vi "Check for Valid File Paths.vi"(8 "error in":errorcluster, 10 "Input Paths (in)":T1={"Golden Template (Source) - (make relative)"=path "E:/Documents/Projects/SPIAPI/Pre-GitHub/Scripting Code 02_10_15 - Cleanup Time/IONode", "Destination Generated Code (make relative)"=path "E:/Documents/Projects/SPIAPI/Pre-GitHub/Scripting Code 02_10_15 - Cleanup Time/Test", "LabVIEW Project to Script"=path "E:/Documents/Projects/SPIAPI/Pre-GitHub/Scripting Code 02_10_15 - Cleanup Time/Test/Test.lvproj", "Placement VI"=path "E:/Documents/Projects/SPIAPI/Pre-GitHub/Scripting Code 02_10_15 - Cleanup Time/Test/TestVI.VI"}, 11 "State Queue In":refnum<queue>) -> (0 "error out":errorcluster, 2 "Inputs Paths (out)":T1={"Golden Template (Source) - (make relative)"=path "E:/Documents/Projects/SPIAPI/Scripting Code  with State Machine 01_12_15 - IO Node Control Still Needs Updating/IONode", "Destination Generated Code (make relative)"=path "E:/Documents/Projects/SPIAPI/Examples", "LabVIEW Project to Script"=path "E:/Documents/Projects/SPIAPI/Examples/SPI Engine Example.lvproj", "Placement VI"=path "E:/Documents/Projects/SPIAPI/Examples/PMOD Example(FPGA).vi"}, 3 "State Queue Out":refnum<queue>)   [LabVIEW 2014]
doc: "Checks if a file/ folder exists at all input paths. Throws an error if they don't. If the Placement VI is blank, change the path to point to Generated Code.vi and queue Generate FPGA VI state.s"
uses:
  Controls/Input Paths.ctl
  Scripting States.ctl
  Initialization and IO Node Scripting.lvlib
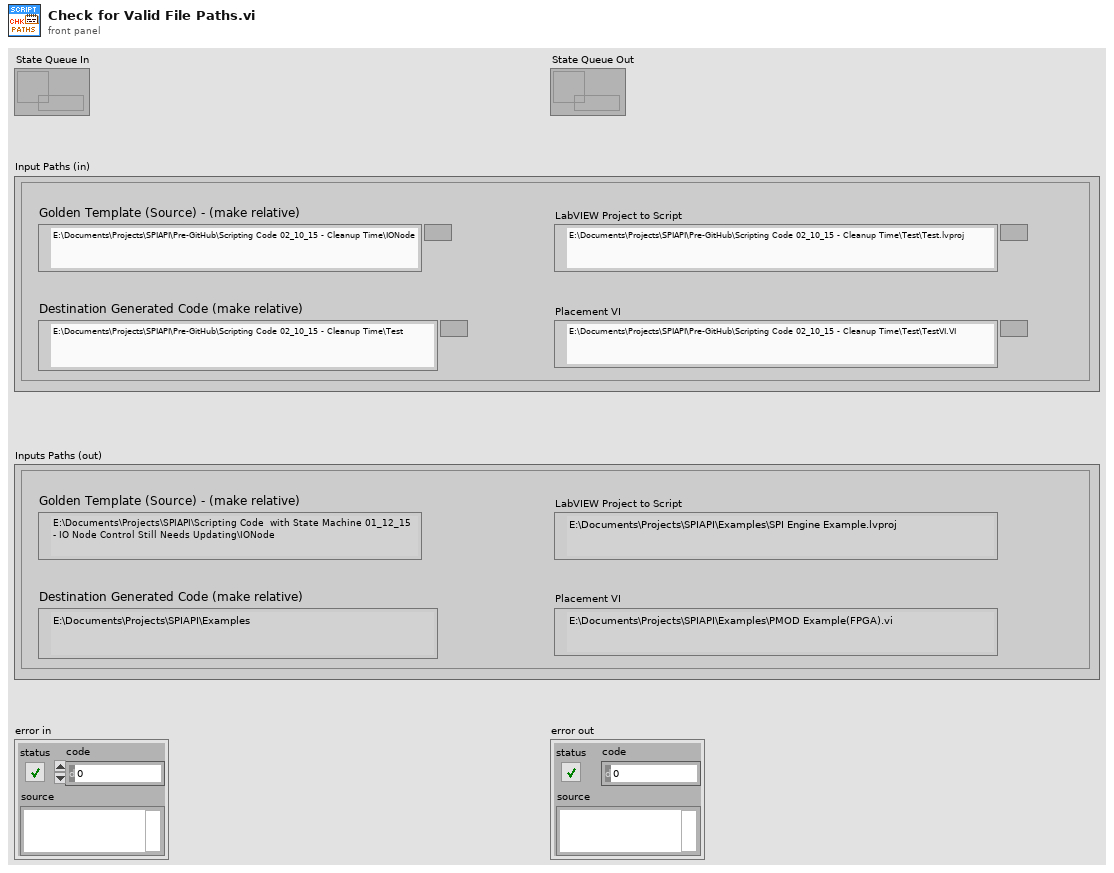
[diagram p1: front panel]
types:
  T1 = typedef "Initialization and IO Node Scripting.lvlib/Input Paths.ctl" = cluster{"Golden Template (Source) - (make relative)":path, "Destination Generated Code (make relative)":path, "LabVIEW Project to Script":path, "Placement VI":path}
  T2 = typedef "Scripting States.ctl" = enum16{"Initialize", "Modify Dequeue Commands", "Modify Enqueue Data", "Create FPGA VI", "Create Project FIFOs", "Create IO Nodes", "Place IO Nodes", "Update Node Count in Engine", "Expand FIFO Type Def", "Populate FIFO Names in Engine", "Modify I/O Pin Names", "Modify I/O Pin Enable", "Replace DLU", "Add Engine to Project", "Place SPI Engine", "Scripting Complete Check", "End"}
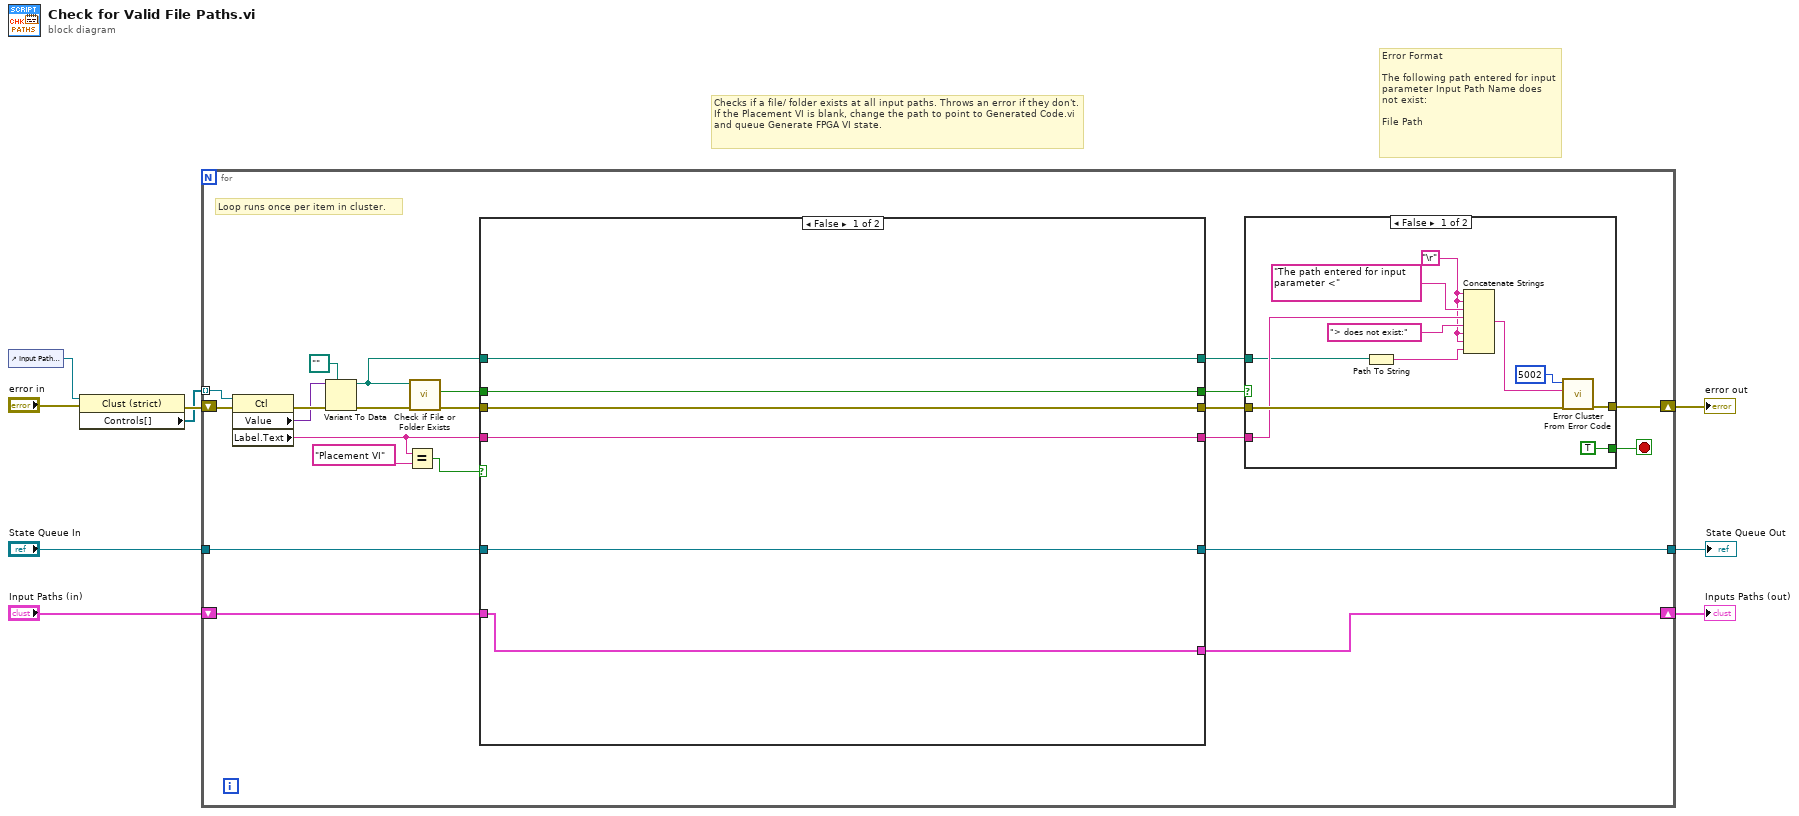
[diagram p0: block diagram]
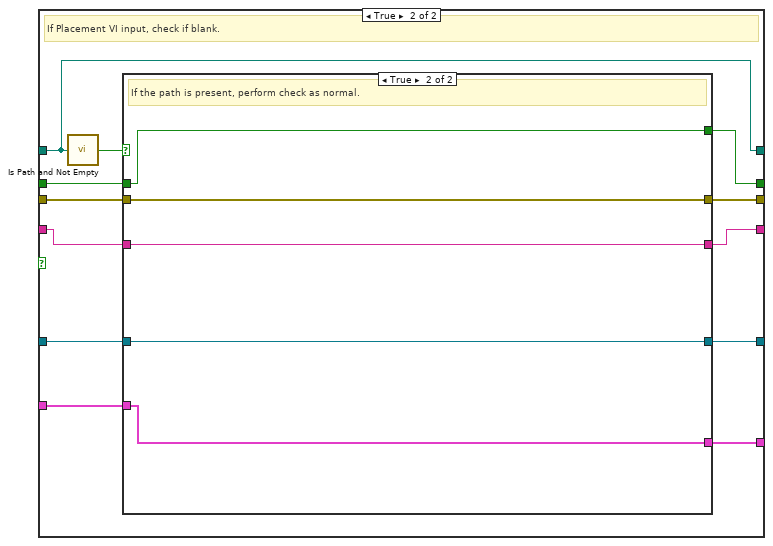
[diagram p2: hidden frame]
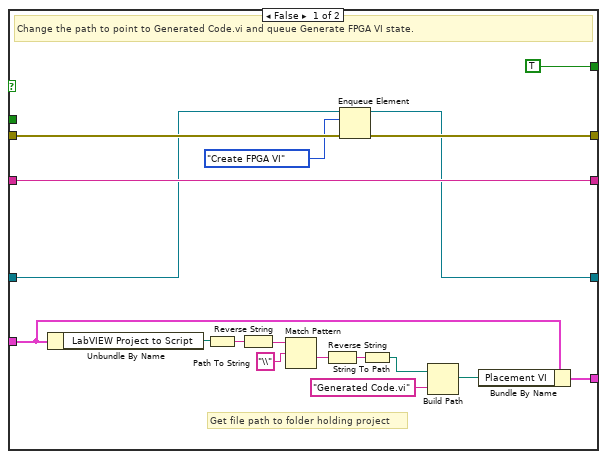
[diagram p3: hidden frame]
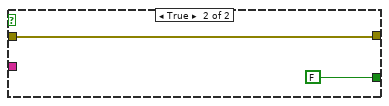
[diagram p4: hidden frame]
diagram:
  # "Error Format\n\nThe following path entered for input parameter Input Path Name does not exist:\n\nFile Path"
  # "Checks if a file/ folder exists at all input paths. Throws an error if they don't. If the Placement VI is blank, change the path to point to Generated Code.vi and queue Generate FPGA VI state."
  n1 = control-ref of="Input Paths (in)"() -> (w5:refnum<vi>)
  n2 = property class="Clust (strict)"(reference=w5, error in="error in") -> (error out=w9:errorcluster, "Controls[]"=w8:refnum<vi>[])  [unwired: 1 out]
  n3 = for {
    tunnel: w8 -> [w30] mode=indexing
    shift-right: [w15] -> w3
    shift-left: "Input Paths (in)" -> [w21]
    shift-right: [w25] -> w6
    shift-left: w9 -> [w31]
    tunnel: "State Queue In" -> [w11]
    tunnel: [w10] -> w1
    stop <- w24 stop-if-true
    # "Loop runs once per item in cluster."
    n4 = property class="Ctl"(reference=w30, error in=w31) -> (error out=w29:errorcluster, "Value"=w26:variant, "Label.Text"=w14:string)  [unwired: 1 out]
    n5 = Variant To Data(error in=w29, type=path "", Variant=w26) -> (data=w20:path, error out=w28:errorcluster)
    n6 = Equal?(x=w14, y="Placement VI" ("x")) -> (x = y?=w23:bool)
    n7 = call <vilib>:"Check if File or Folder Exists.vi"("error in (no error)"=w28, "path"=w20) -> ("error out"=w16:errorcluster, "file or folder exists?"=w18:bool)  [unwired: 7 in, 1 out]
    n8 = case shown="False" w23 {
      tunnel: w21 -> [w34 w48]
      tunnel: [w37 w47] -> w19
      tunnel: w20 -> [w37 w47]
      tunnel: [w35 w40] -> w12
      tunnel: w18 -> [w35 w41]
      tunnel: [w36 w45] -> w17
      tunnel: w16 -> [w36 w46]
      tunnel: [w34 w44] -> w15
      tunnel: [w33 w42] -> w13
      tunnel: w14 -> [w33 w43]
      tunnel: w11 -> [w32 w39]
      tunnel: [w32 w38] -> w10
      frame False {
      }
      frame True {
        # "If Placement VI input, check if blank."
        n9 = call <vilib>:"Is Path and Not Empty.vi"("path"=w47) -> ("Is Path and Not Empty?"=w49:bool)  [unwired: 4 in]
        n10 = case shown="True" w49 {
          tunnel: [w58 w72] -> w44
          tunnel: w48 -> [w57 w72]
          tunnel: w46 -> [w56 w71]
          tunnel: [w55 w71] -> w45
          tunnel: [w53 w70] -> w42
          tunnel: w43 -> [w53 w70]
          tunnel: w41 -> [_ w69]
          tunnel: [TRUE ("file or folder exists?") w69] -> w40
          tunnel: w39 -> [w51 w68]
          tunnel: [w50 w68] -> w38
          frame False {
            # "Get file path to folder holding project"
            # "Change the path to point to Generated Code.vi and queue Generate FPGA VI state."
            n11 = Unbundle By Name(w57) -> ("LabVIEW Project to Script"=w62:path)
            n12 = Path To String(path=w62) -> (string=w67:string)
            n13 = Reverse String(1:w67) -> (0:w66:string)
            n14 = Match Pattern(string=w66, regular expression="\\") -> (after substring=w65:string)  [unwired: 1 in, 3 out]
            n15 = Reverse String(1:w65) -> (0:w63:string)
            n16 = Enqueue Element(queue=w51, element=Scripting_States."Create FPGA VI", error in (no error)=w56) -> (queue out=w50:refnum<queue>, error out=w55:errorcluster)  [unwired: 1 in, 1 out]
            n17 = String To Path(string=w63) -> (path=w60:path)
            n18 = Build Path(base path=w60, name or relative path="Generated Code.vi") -> (appended path=w59:path)
            n19 = Bundle By Name(cluster=w57, "Placement VI"=w59) -> (w58:T1)
          }
          frame True {
            # "If the path is present, perform check as normal."
          }
        }
      }
    }
    n20 = case shown="False" w12 {
      tunnel: w17 -> [w83 w85]
      tunnel: w13 -> [w77 _]
      tunnel: [w80 w85] -> w25
      tunnel: [TRUE FALSE] -> w24
      tunnel: w19 -> [w73 _]
      frame False {
        w74 = "\r"
        n21 = Path To String(path=w73) -> (string=w75:string)
        n22 = Concatenate Strings(w74, w74, "The path entered for input parameter <" ("string"), w77, "> does not exist:" ("string"), w74, w74, w75) -> (w82:string)
        n23 = call <vilib>:"Error Cluster From Error Code.vi"("error in (no error)"=w83, "error message (\"\")"=w82, "error code (0)"=5002) -> ("error out"=w80:errorcluster)  [unwired: 6 in]
      }
      frame True {
      }
    }
  }
  "error out" <- w6
  "Inputs Paths (out)" <- w3
  "State Queue Out" <- w1
